vi "SetBits.vi"(8 "Datain":u8, 9 "Pos":u8, 10 "Mask":u8, 11 "Reg data":u16) -> (2 "Data":u16)   [LabVIEW 2022 SP3, in "BME680.lvlib" / "BME680.lvclass"]
uses:
  BME680.lvclass
  BME680.lvclass/BME680.ctl
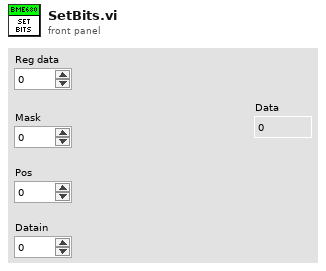
[diagram p1: front panel]
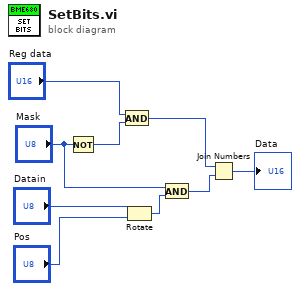
[diagram p0: block diagram]
diagram:
  n1 = Not(x="Mask") -> (.not. x?=w8:u8)
  n2 = And(x="Reg data", y=w8) -> (x .and. y?=w3:u16)
  n3 = Rotate(1:"Pos", 2:"Datain") -> (0:w4:u8)
  n4 = And(x="Mask", y=w4) -> (x .and. y?=w2:u8)
  n5 = Join Numbers(hi=w3, lo=w2) -> ((hi.lo)=→"Data":u32)
